vi "VSG25A_StepSweep.vi"(0 "Device Handle In":i32, 1 "Run as Subpanel":bool, 2 "RampSweep Cluster In":T1={"Start Freq"=990.0, "Stop Freq"=1010.0, "Start Hz"=2, "Stop Hz"=2, "Sweep Time"=10.0, "Amplitude"=-80.0, "Sweep Factor (sec)"=5} {"Sweep Factor (sec)" items=["tera", "giga", "Mega", "kilo", "unity", "milli", "micro", "nano", "pico"]; "Start Hz" items=["Hz", "kHz", "MHz", "GHz"]; "Stop Hz" items=["Hz", "kHz", "MHz", "GHz"]}, 3 "Error In":errorcluster) -> (5 "Device Handle Out":i32, 6 "RampSweep Cluster Out":T1 {"Sweep Factor (sec)" items=["tera", "giga", "Mega", "kilo", "unity", "milli", "micro", "nano", "pico"]; "Start Hz" items=["Hz", "kHz", "MHz", "GHz"]; "Stop Hz" items=["Hz", "kHz", "MHz", "GHz"]}, 7 "Error Out":errorcluster)   [LabVIEW 2014]
uses:
  Controls/Frequency Hertz.ctl
  Controls/Sweep Cluster.ctl
  Controls/Factor Control.ctl
  Controls/Ramp Sweep Write Steps.ctl
  sg_lib/VSG25A.lvlib
panel:
  in  "Sweep Factor \n(Seconds)":T3 items=["tera", "giga", "Mega", "kilo", "unity", "milli", "micro", "nano", "pico"]
  out "Frequency Span":dbl
  in  "Stop":bool
  out "Device Selected":bool
  in  "Sweep Time":dbl
  in  "Stop Hz":T2 items=["Hz", "kHz", "MHz", "GHz"]
  in  "Stop Frequency":dbl
  in  "RF On":bool
  in  "Start Hz":T2 items=["Hz", "kHz", "MHz", "GHz"]
  in  "Amplitude (dBm)":dbl
  in  "Start Frequency":dbl
  # "Step Sweep"
  # "(<= 10/Span)"
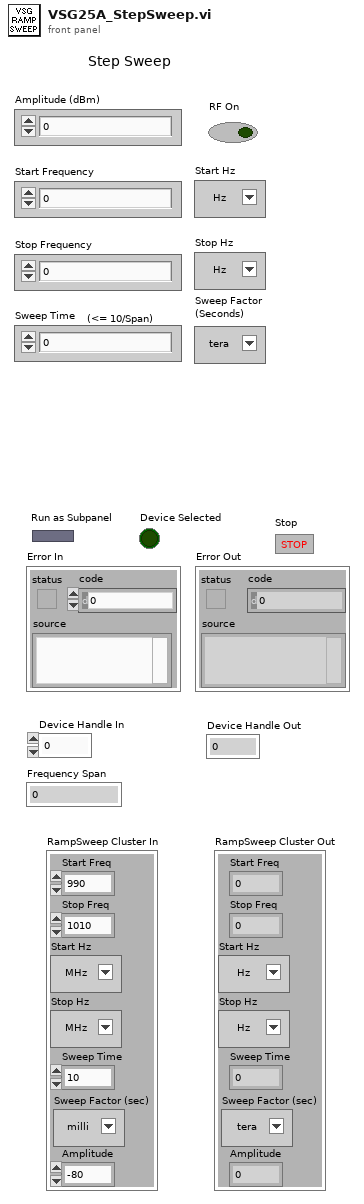
[diagram p1: front panel]
types:
  T1 = typedef "Sweep Cluster.ctl" = cluster{"Start Freq":dbl, "Stop Freq":dbl, "Start Hz":T2, "Stop Hz":T2, "Sweep Time":dbl, "Amplitude":dbl, "Sweep Factor (sec)":T3}
  T2 = typedef "Frequency Hertz.ctl" = u16
  T3 = typedef "Factor Control.ctl" = u16
  T4 = enum16{"Init", "Proc Events", "Write VSG25", "Exit"}
  T5 = enum32{"Bad", "Idle", "Run top level", "Running"}
  T6 = typedef "Ramp Sweep Write Steps.ctl" = enum16{"Check Amplitude", "Check Start Freq", "Check Stop Freq", "Check Sweep Time", "Calc Freq Span", "Stop RF", "Set Freq And Amp", "Set Sweep", "Finish", ""}
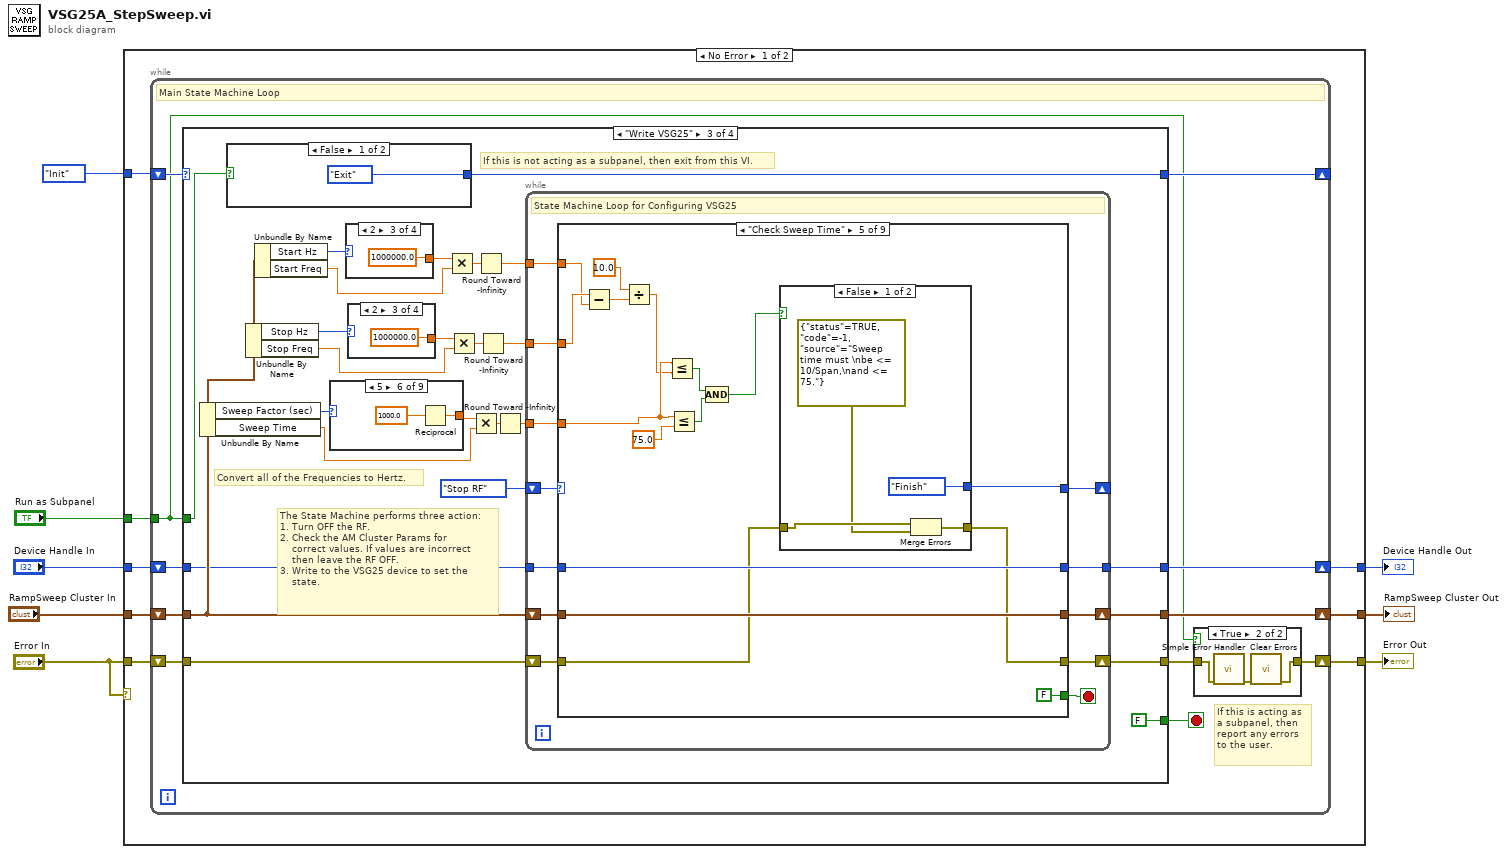
[diagram p0: block diagram]
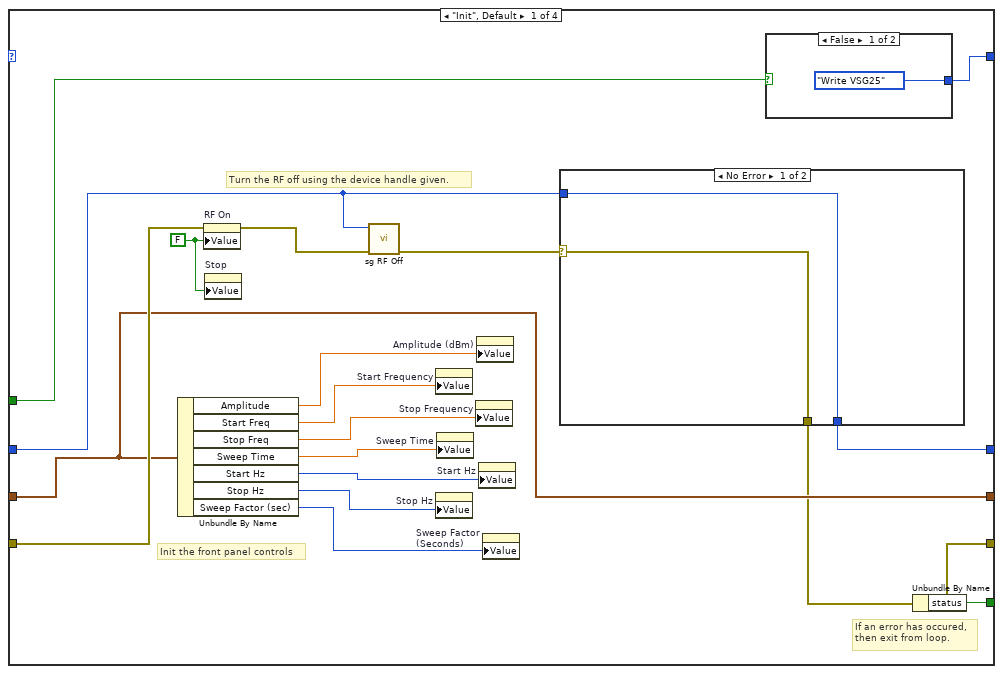
[diagram p3: hidden frame]
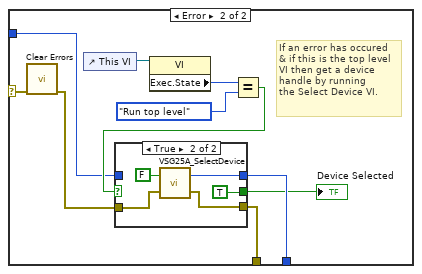
[diagram p4: hidden frame]
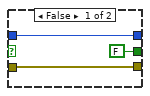
[diagram p5: hidden frame]
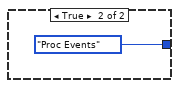
[diagram p6: hidden frame]
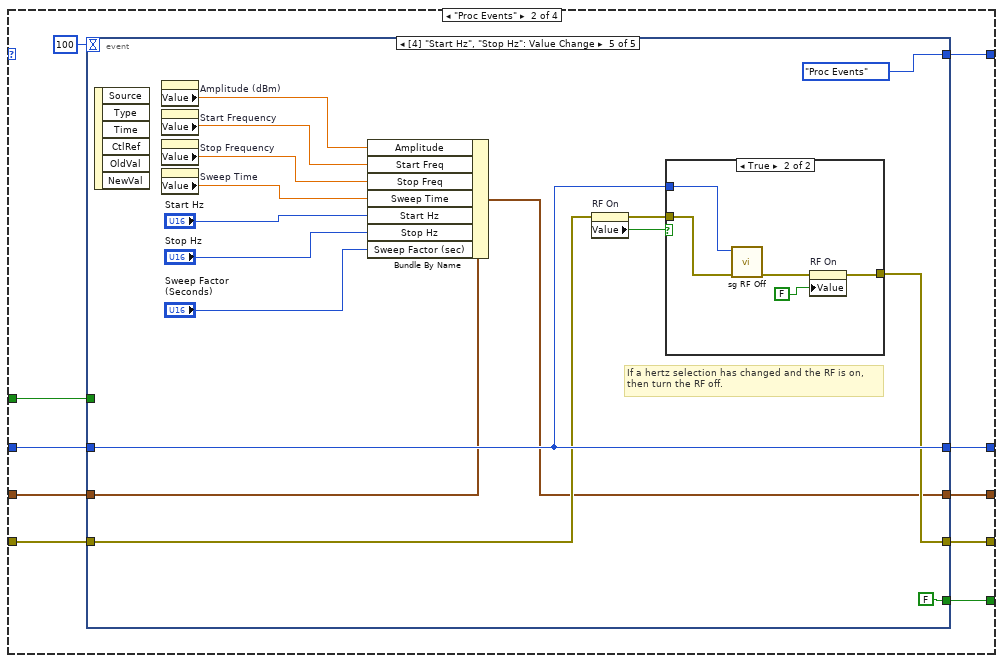
[diagram p7: hidden frame]
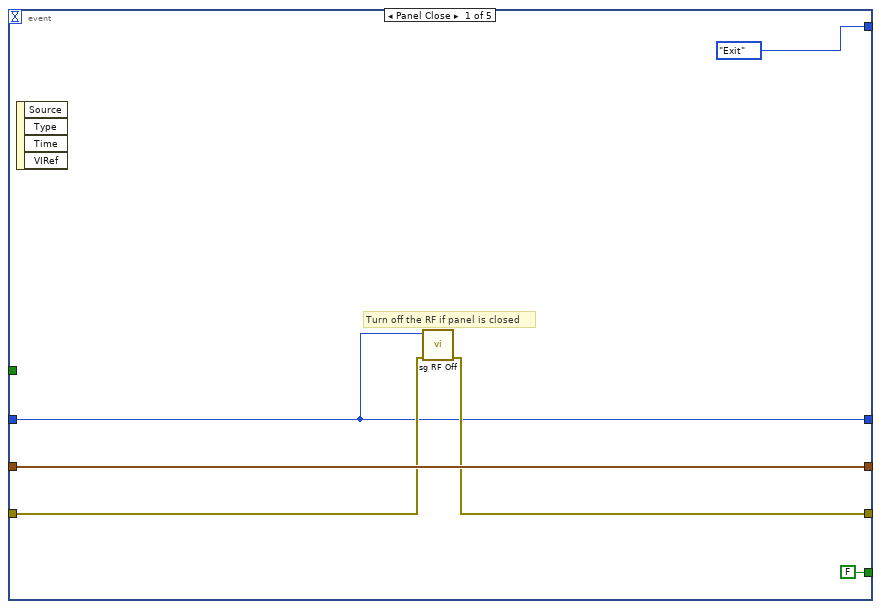
[diagram p8: hidden frame]
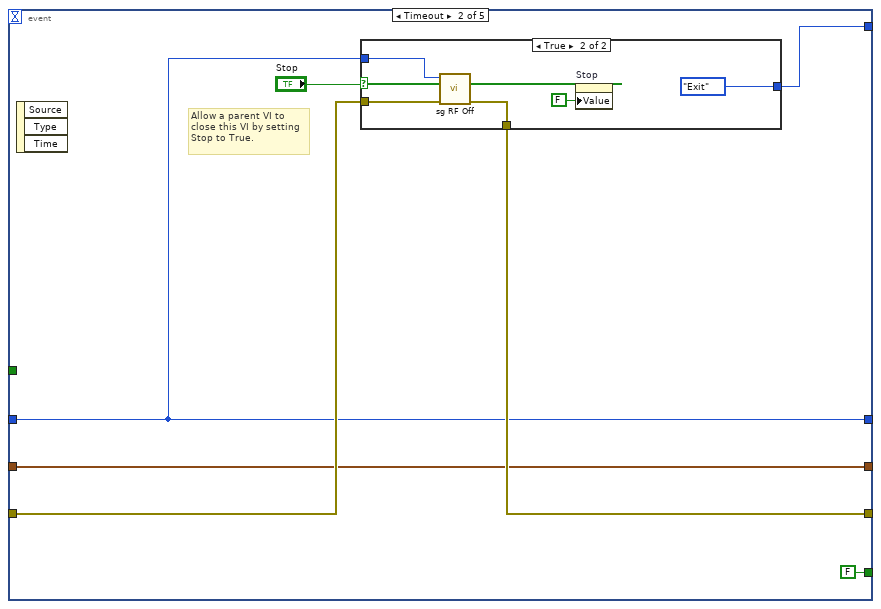
[diagram p9: hidden frame]
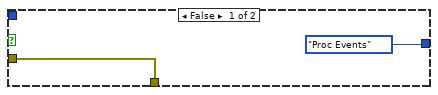
[diagram p10: hidden frame]
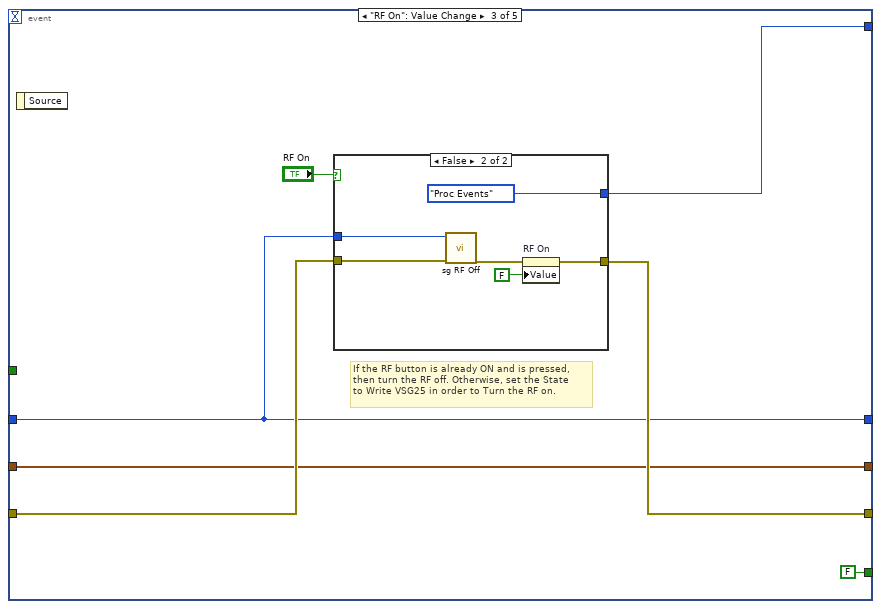
[diagram p11: hidden frame]
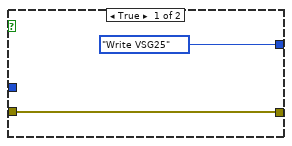
[diagram p12: hidden frame]
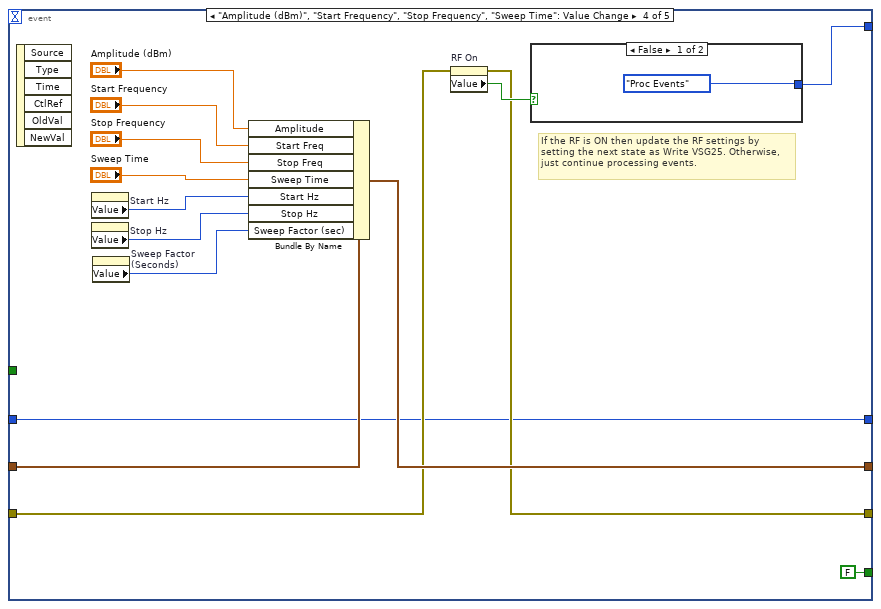
[diagram p13: hidden frame]
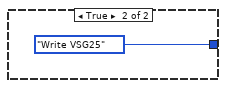
[diagram p14: hidden frame]
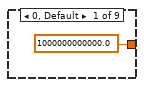
[diagram p16: hidden frame]
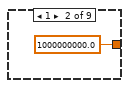
[diagram p17: hidden frame]
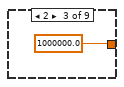
[diagram p18: hidden frame]
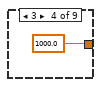
[diagram p19: hidden frame]
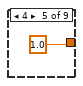
[diagram p20: hidden frame]
diagram:
  n1 = case shown="No Error" "Error In" {
    tunnel: "Error In" -> [w12 w360]
    tunnel: T4."Init" -> [w16 _]
    tunnel: "Run as Subpanel" -> [w15 _]
    tunnel: "Device Handle In" -> [w14 w358]
    tunnel: "RampSweep Cluster In" -> [w13 w359]
    tunnel: [w11 w360] -> w4
    tunnel: [w10 w359] -> w2
    tunnel: [w9 w358] -> w3
    frame No Error {
      n2 = while {
        shift-right: [w26] -> _
        shift-left: w16 -> [w27]
        tunnel: w15 -> [w17]
        shift-right: [w18] -> w11
        shift-left: w12 -> [w23]
        shift-right: [w21] -> w10
        shift-left: w13 -> [w24]
        shift-right: [w20] -> w9
        shift-left: w14 -> [w25]
        stop <- w22 stop-if-true
        # "If this is acting as \na subpanel, then\nreport any errors\nto the user."
        # "Main State Machine Loop"
        n3 = case shown="\"Write VSG25\"" w27 {
          selector: w27 -> [_ _ _ w353]
          tunnel: [w42 w74 w161 w353] -> w26
          tunnel: w17 -> [w45 w78 w160 _]
          tunnel: w25 -> [w36 w79 w166 w348]
          tunnel: w24 -> [w43 w80 w167 w349]
          tunnel: w23 -> [w44 w81 w171 w350]
          tunnel: [w41 w75 FALSE TRUE] -> w22
          tunnel: [w37 w73 w165 w351] -> w19
          tunnel: [w43 w77 w164 w349] -> w21
          tunnel: [w38 w76 w163 w348] -> w20
          frame "Init", Default {
            w35 = FALSE ("RF On")
            # "Init the front panel controls"
            # "Turn the RF off using the device handle given."
            # "If an error has occured,\nthen exit from loop."
            n4 = Unbundle By Name(w43) -> ("Amplitude"=w49:dbl, "Start Freq"=w48:dbl, "Stop Freq"=w47:dbl, "Sweep Time"=w46:dbl, "Start Hz"=w34:T2, "Stop Hz"=w33:T2, "Sweep Factor (sec)"=w32:T3)
            n5 = property on="RF On" class="Bool (strict)"(error in=w44, "Value"=w35) -> (error out=w40:errorcluster)  [unwired: 1 in, 1 out]
            n6 = property on="Stop" class="Bool (strict)"("Value"=w35) -> ()  [unwired: 2 in, 2 out]
            n7 = call "sg RF Off.vi"("error in (no error)"=w40, "device"=w36) -> ("error out"=w39:errorcluster)  [unwired: 8 in, 1 out]
            n8 = property on="Start Frequency" class="DigNum (strict)"("Value"=w48) -> ()  [unwired: 2 in, 2 out]
            n9 = property on="Stop Hz" class="Ring (strict)"("Value"=w33) -> ()  [unwired: 2 in, 2 out]
            n10 = property on="Sweep Time" class="DigNum (strict)"("Value"=w46) -> ()  [unwired: 2 in, 2 out]
            n11 = property on="Stop Frequency" class="DigNum (strict)"("Value"=w47) -> ()  [unwired: 2 in, 2 out]
            n12 = property on="Amplitude (dBm)" class="DigNum (strict)"("Value"=w49) -> ()  [unwired: 2 in, 2 out]
            n13 = property on="Start Hz" class="Ring (strict)"("Value"=w34) -> ()  [unwired: 2 in, 2 out]
            n14 = property on="Sweep Factor \n(Seconds)" class="Ring (strict)"("Value"=w32) -> ()  [unwired: 2 in, 2 out]
            n15 = case shown="No Error" w39 {
              selector: w39 -> [w50 w57]
              tunnel: [w51 w55] -> w38
              tunnel: [w50 w54] -> w37
              tunnel: w36 -> [w51 w53]
              frame No Error {
              }
              frame Error {
                # "If an error has occured\n& if this is the top level\nVI then get a device\nhandle by running \nthe Select Device VI."
                n16 = call <vilib>:"Clear Errors.vi"("error in (no error)"=w57) -> ("error out"=w56:errorcluster)  [unwired: 5 in, 1 out]
                n17 = control-ref of="This VI"() -> (w61:refnum<vi>)
                n18 = property class="VI"(reference=w61) -> ("Exec.State"=w60:T5)  [unwired: 1 in, 2 out]
                n19 = Equal?(x=w60, y=T5."Run top level" ("Execution:State 2")) -> (x = y?=w58:bool)
                n20 = case shown="True" w58 {
                  tunnel: [w64 w69] -> w55
                  tunnel: w53 -> [w64 _]
                  tunnel: w56 -> [w63 w67]
                  tunnel: [w63 w66] -> w54
                  tunnel: [FALSE TRUE] -> w52
                  frame False {
                  }
                  frame True {
                    n21 = call "VSG25A_SelectDevice.vi"("ErrorIn"=w67, "AutoSel"=FALSE) -> ("ErrorOut"=w66:errorcluster, "deviceHandle"=w69:i32)
                  }
                }
                "Device Selected" <- w52
              }
            }
            n22 = case shown="False" w45 {
              tunnel: [T4."Write VSG25" T4."Proc Events"] -> w42
              frame False {
              }
              frame True {
              }
            }
            n23 = Unbundle By Name(w37) -> ("status"=w41:bool)
          }
          frame "Proc Events" {
            n24 = event shown="[4] \"Start Hz\", \"Stop Hz\": Value Change" {
              selector: _ -> [_ _ _ _ _]
              dyn-events: _ -> [_ _ _ _ _]
              timeout: 100 -> [_ _ _ _ _]
              tunnel: w81 -> [w84 w91 w107 w123 w145]
              tunnel: w80 -> [w85 w89 w105 w131 w144]
              tunnel: w79 -> [w82 w88 w104 w121 w147]
              tunnel: w78 -> [_ _ _ _ _]
              tunnel: [w83 w90 w106 w122 w146] -> w73
              tunnel: [w85 w89 w105 w130 w143] -> w77
              tunnel: [w82 w88 w104 w121 w147] -> w76
              tunnel: [FALSE FALSE FALSE FALSE FALSE] -> w75
              tunnel: [T4."Exit" w92 w103 w124 T4."Proc Events"] -> w74
              event Panel Close {
                # "Turn off the RF if panel is closed"
                n25 = event-data() -> ()  [unwired: 1 in, 4 out]
                n26 = call "sg RF Off.vi"("error in (no error)"=w84, "device"=w82) -> ("error out"=w83:errorcluster)  [unwired: 8 in, 1 out]
              }
              event Timeout {
                # "Allow a parent VI to \nclose this VI by setting\nStop to True."
                n27 = event-data() -> ()  [unwired: 1 in, 3 out]
                n28 = case shown="True" "Stop" {
                  tunnel: [T4."Proc Events" T4."Exit"] -> w92
                  tunnel: w91 -> [w95 w100]
                  tunnel: [w95 w99] -> w90
                  tunnel: w88 -> [_ w98]
                  frame False {
                  }
                  frame True {
                    n29 = call "sg RF Off.vi"("error in (no error)"=w100, "device"=w98) -> ("error out"=w99:errorcluster)  [unwired: 8 in, 1 out]
                    n30 = property on="Stop" class="Bool (strict)"("Value"=FALSE ("Stop")) -> ()  [unwired: 2 in, 2 out]
                  }
                }
              }
              event "RF On": Value Change {
                # "If the RF button is already ON and is pressed, \nthen turn the RF off. Otherwise, set the State\nto Write VSG25 in order to Turn the RF on."
                n31 = event-data() -> ()  [unwired: 1 in, 1 out]
                n32 = case shown="False" "RF On" {
                  tunnel: [w109 w114] -> w106
                  tunnel: w107 -> [w109 w116]
                  tunnel: w104 -> [_ w115]
                  tunnel: [T4."Write VSG25" T4."Proc Events"] -> w103
                  frame True {
                  }
                  frame False {
                    n33 = call "sg RF Off.vi"("error in (no error)"=w116, "device"=w115) -> ("error out"=w113:errorcluster)  [unwired: 8 in, 1 out]
                    n34 = property on="RF On" class="Bool (strict)"(error in=w113, "Value"=FALSE ("RF On")) -> (error out=w114:errorcluster)  [unwired: 1 in, 1 out]
                  }
                }
              }
              event "Amplitude (dBm)", "Start Frequency", "Stop Frequency", "Sweep Time": Value Change {
                # "If the RF is ON then update the RF settings by\nsetting the next state as Write VSG25. Otherwise,\njust continue processing events."
                n35 = event-data() -> ()  [unwired: 1 in, 6 out]
                n36 = property on="Start Hz" class="Ring (strict)"() -> ("Value"=w119:T2)  [unwired: 2 in, 2 out]
                n37 = property on="Stop Hz" class="Ring (strict)"() -> ("Value"=w118:T2)  [unwired: 2 in, 2 out]
                n38 = property on="Sweep Factor \n(Seconds)" class="Ring (strict)"() -> ("Value"=w117:T3)  [unwired: 2 in, 2 out]
                n39 = Bundle By Name(cluster=w131, "Amplitude"="Amplitude (dBm)", "Start Freq"="Start Frequency", "Stop Freq"="Stop Frequency", "Sweep Time"="Sweep Time", "Start Hz"=w119, "Stop Hz"=w118, "Sweep Factor (sec)"=w117) -> (w130:T1)
                n40 = property on="RF On" class="Bool (strict)"(error in=w123) -> (error out=w122:errorcluster, "Value"=w125:bool)  [unwired: 1 in, 1 out]
                n41 = case shown="False" w125 {
                  tunnel: [T4."Proc Events" T4."Write VSG25"] -> w124
                  frame False {
                  }
                  frame True {
                  }
                }
              }
              event Value Change {
                # "If a hertz selection has changed and the RF is on,\nthen turn the RF off."
                n42 = event-data() -> ()  [unwired: 1 in, 6 out]
                n43 = property on="Amplitude (dBm)" class="DigNum (strict)"() -> ("Value"=w142:dbl)  [unwired: 2 in, 2 out]
                n44 = property on="Start Frequency" class="DigNum (strict)"() -> ("Value"=w141:dbl)  [unwired: 2 in, 2 out]
                n45 = property on="Stop Frequency" class="DigNum (strict)"() -> ("Value"=w140:dbl)  [unwired: 2 in, 2 out]
                n46 = property on="Sweep Time" class="DigNum (strict)"() -> ("Value"=w139:dbl)  [unwired: 2 in, 2 out]
                n47 = Bundle By Name(cluster=w144, "Amplitude"=w142, "Start Freq"=w141, "Stop Freq"=w140, "Sweep Time"=w139, "Start Hz"="Start Hz", "Stop Hz"="Stop Hz", "Sweep Factor (sec)"="Sweep Factor \n(Seconds)") -> (w143:T1)
                n48 = property on="RF On" class="Bool (strict)"(error in=w145) -> (error out=w149:errorcluster, "Value"=w148:bool)  [unwired: 1 in, 1 out]
                n49 = case shown="True" w148 {
                  tunnel: [w150 w151] -> w146
                  tunnel: w149 -> [w150 w155]
                  tunnel: w147 -> [_ w154]
                  frame False {
                  }
                  frame True {
                    n50 = call "sg RF Off.vi"("error in (no error)"=w155, "device"=w154) -> ("error out"=w152:errorcluster)  [unwired: 8 in, 1 out]
                    n51 = property on="RF On" class="Bool (strict)"(error in=w152, "Value"=FALSE ("RF On")) -> (error out=w151:errorcluster)  [unwired: 1 in, 1 out]
                  }
                }
              }
            }
          }
          frame "Write VSG25" {
            # "If this is not acting as a subpanel, then exit from this VI."
            # "Convert all of the Frequencies to Hertz."
            # "The State Machine performs three action:\n1. Turn OFF the RF.\n2. Check the AM Cluster Params for \n    correct values. If values are incorrect\n    then leave the RF OFF.\n3. Write to the VSG25 device to set the\n    state."
            n52 = Unbundle By Name(w167) -> ("Sweep Factor (sec)"=w159:T3, "Sweep Time"=w158:dbl)
            n53 = case shown="False" w160 {
              tunnel: [T4."Exit" T4."Proc Events"] -> w161
              frame False {
              }
              frame True {
              }
            }
            n54 = Unbundle By Name(w167) -> ("Stop Hz"=w174:T2, "Stop Freq"=w176:dbl)
            n55 = Unbundle By Name(w167) -> ("Start Hz"=w179:T2, "Start Freq"=w177:dbl)
            n56 = case shown="5" w159 {
              tunnel: [1000000000000.0 1000000000.0 ("y") 1000000.0 ("y") 1000.0 ("y") 1.0 ("y") w187 w189 w191 w193] -> w157
              frame 0, Default {
              }
              frame 1 {
              }
              frame 2 {
              }
              frame 3 {
              }
              frame 4 {
              }
              frame 5 {
                n57 = Reciprocal(x=1000.0 ("y")) -> (1/x=w187:dbl)
              }
              frame 6 {
                n58 = Reciprocal(x=1000000.0 ("y")) -> (1/x=w189:dbl)
              }
              frame 7 {
                n59 = Reciprocal(x=1000000000.0 ("y")) -> (1/x=w191:dbl)
              }
              frame 8 {
                n60 = Reciprocal(x=1000000000000.0) -> (1/x=w193:dbl)
              }
            }
            n61 = case shown="2" w179 {
              tunnel: [1.0 ("y") 1000.0 ("y") 1000000.0 ("y") 1000000000.0 ("y")] -> w178
              frame 0, Default {
              }
              frame 1 {
              }
              frame 2 {
              }
              frame 3 {
              }
            }
            n62 = case shown="2" w174 {
              tunnel: [1.0 ("y") 1000.0 ("y") 1000000.0 ("y") 1000000000.0 ("y")] -> w175
              frame 0, Default {
              }
              frame 1 {
              }
              frame 2 {
              }
              frame 3 {
              }
            }
            n63 = Multiply(x=w178, y=w177) -> (x*y=w180:dbl)
            n64 = Multiply(x=w175, y=w176) -> (x*y=w173:dbl)
            n65 = Multiply(x=w157, y=w158) -> (x*y=w172:dbl)
            n66 = Round Toward -Infinity(1:w180) -> (0:w170:dbl)
            n67 = Round Toward -Infinity(1:w173) -> (0:w169:dbl)
            n68 = Round Toward -Infinity(1:w172) -> (0:w168:dbl)
            n69 = while {
              tunnel: w170 -> [w210]
              tunnel: w169 -> [w209]
              tunnel: w168 -> [w208]
              tunnel: w166 -> [w206]
              tunnel: [w203] -> w163
              shift-right: [w205] -> w165
              shift-left: w171 -> [w211]
              shift-right: [w204] -> w164
              shift-left: w167 -> [w207]
              shift-right: [w200] -> _
              shift-left: Ramp_Sweep_Write_Steps."Stop RF" -> [w201]
              stop <- w202 stop-if-true
              # "State Machine Loop for Configuring VSG25"
              n70 = case shown="\"Check Sweep Time\"" w201 {
                selector: w201 -> [_ _ _ _ _ _ _ _ w335]
                tunnel: w211 -> [w217 w220 w257 w275 w297 w310 w325 w334 w336]
                tunnel: w210 -> [_ _ w248 _ w290 w309 w317 _ _]
                tunnel: w209 -> [_ _ w247 w269 w291 w308 _ _ _]
                tunnel: w208 -> [_ _ _ _ w287 _ _ w327 _]
                tunnel: w207 -> [w215 w224 w258 w277 w299 w314 w323 w332 w337]
                tunnel: w206 -> [w214 w222 w259 w276 w298 w313 w322 w331 w338]
                tunnel: [w216 w219 w256 w274 w296 w310 w324 w333 w336] -> w205
                tunnel: [w215 w223 w258 w277 w299 w314 w323 w332 w337] -> w204
                tunnel: [w214 w222 w259 w276 w298 w313 w322 w331 w338] -> w203
                tunnel: [FALSE FALSE FALSE FALSE FALSE FALSE FALSE FALSE TRUE] -> w202
                tunnel: [Ramp_Sweep_Write_Steps."Check Amplitude" w218 w250 w267 w292 Ramp_Sweep_Write_Steps."Set Freq And Amp" Ramp_Sweep_Write_Steps."Set Sweep" Ramp_Sweep_Write_Steps."Finish" w335] -> w200
                frame "Stop RF", Default {
                  n71 = call "sg RF Off.vi"("error in (no error)"=w217, "device"=w214) -> ("error out"=w216:errorcluster)  [unwired: 8 in, 1 out]
                }
                frame "Check Amplitude" {
                  n72 = Unbundle By Name(w224) -> ("Amplitude"=w230:dbl)
                  n73 = Less Or Equal?(x=w230, y=10.0) -> (x <= y?=w226:bool)
                  n74 = Greater Or Equal?(x=w230, y=-80.0) -> (x >= y?=w229:bool)
                  n75 = And(x=w226, y=w229) -> (x .and. y?=w225:bool)
                  n76 = case shown="True" w225 {
                    tunnel: w229 -> [w240 _]
                    tunnel: w230 -> [_ w245]
                    tunnel: w224 -> [w237 w244]
                    tunnel: [w236 w243] -> w223
                    tunnel: w220 -> [w234 w242]
                    tunnel: [w232 w242] -> w219
                    tunnel: [Ramp_Sweep_Write_Steps."Finish" Ramp_Sweep_Write_Steps."Check Start Freq"] -> w218
                    frame False {
                      n77 = Select(t=10.0, s=w240, f=-80.0) -> (s? t:f=w235:dbl)
                      n78 = Bundle By Name(cluster=w237, "Start Freq"=w235) -> (w236:T1)
                      n79 = property on="Amplitude (dBm)" class="DigNum (strict)"("Value"=w235) -> ()  [unwired: 2 in, 2 out]
                      n80 = Merge Errors(w234, errorcluster {"status"=TRUE, "code"=-1, "source"="Invalid Amplitude.\nValue must be between\n-80 dBm and 10 dBm."} ("error constant")) -> (w232:errorcluster)
                    }
                    frame True {
                      n81 = Round Toward -Infinity(1:w245) -> (0:w246:dbl)
                      n82 = Bundle By Name(cluster=w244, "Amplitude"=w246) -> (w243:T1)
                    }
                  }
                }
                frame "Check Start Freq" {
                  n83 = Greater Or Equal?(x=w248, y=80000000.0) -> (x >= y?=w254:bool)
                  n84 = Less?(x=w248, y=w247) -> (x < y?=w249:bool)
                  n85 = Less Or Equal?(x=w248, y=2500000000.0) -> (x <= y?=w255:bool)
                  n86 = Compound Arithmetic op=AND(w254, w249, w255) -> (w251:bool)
                  n87 = case shown="True" w251 {
                    tunnel: w257 -> [w263 w266]
                    tunnel: [w264 w266] -> w256
                    tunnel: [Ramp_Sweep_Write_Steps."Finish" Ramp_Sweep_Write_Steps."Check Stop Freq"] -> w250
                    frame False {
                      n88 = Merge Errors(w263, errorcluster {"status"=TRUE, "code"=-1, "source"="Start frequency must \nbe greater than 80 MHz,\nless than 2.5 GHz and \nless than stop frequency."} ("error constant")) -> (w264:errorcluster)
                    }
                    frame True {
                    }
                  }
                }
                frame "Check Stop Freq" {
                  n89 = Greater Or Equal?(x=w269, y=80000000.0) -> (x >= y?=w272:bool)
                  n90 = Less Or Equal?(x=w269, y=2500000000.0) -> (x <= y?=w273:bool)
                  n91 = Compound Arithmetic op=AND(w272, w273) -> (w268:bool)
                  n92 = case shown="True" w268 {
                    tunnel: w275 -> [w282 w284]
                    tunnel: [w280 w284] -> w274
                    tunnel: [Ramp_Sweep_Write_Steps."Finish" Ramp_Sweep_Write_Steps."Check Sweep Time"] -> w267
                    frame False {
                      n93 = Merge Errors(w282, errorcluster {"status"=TRUE, "code"=-1, "source"="Stop frequency must \nbe greater than 80 MHz,\nand less than 2.5 GHz."} ("error constant")) -> (w280:errorcluster)
                    }
                    frame True {
                    }
                  }
                }
                frame "Check Sweep Time" {
                  n94 = Subtract(x=w291, y=w290) -> (x-y=w288:dbl)
                  n95 = Divide(x=10.0, y=w288) -> (x/y=w286:dbl)
                  n96 = Less Or Equal?(x=w287, y=w286) -> (x <= y?=w285:bool)
                  n97 = Less Or Equal?(x=w287, y=75.0) -> (x <= y?=w295:bool)
                  n98 = Compound Arithmetic op=AND(w285, w295) -> (w293:bool)
                  n99 = case shown="False" w293 {
                    tunnel: w297 -> [w303 w306]
                    tunnel: [w304 w306] -> w296
                    tunnel: [Ramp_Sweep_Write_Steps."Finish" Ramp_Sweep_Write_Steps."Calc Freq Span"] -> w292
                    frame False {
                      n100 = Merge Errors(w303, errorcluster {"status"=TRUE, "code"=-1, "source"="Sweep time must \nbe <= 10/Span,\nand <= 75."} ("error constant")) -> (w304:errorcluster)
                    }
                    frame True {
                    }
                  }
                }
                frame "Calc Freq Span" {
                  n101 = Subtract(x=w308, y=w309) -> (x-y=→"Frequency Span":dbl)
                }
                frame "Set Freq And Amp" {
                  # "Specify the center frequency of the freq span."
                  n102 = property on="Frequency Span" class="DigNum (strict)"() -> ("Value"=w318:dbl)  [unwired: 2 in, 2 out]
                  n103 = Divide(x=w318, y=2.0) -> (x/y=w320:dbl)
                  n104 = Unbundle By Name(w323) -> ("Amplitude"=w326:dbl)
                  n105 = Add(x=w317, y=w320) -> (x+y=w316:dbl)
                  n106 = call "sg Set Frequency Amplitude.vi"("error in (no error)"=w325, "amplitude"=w326, "frequency"=w316, "device"=w322) -> ("error out"=w324:errorcluster)  [unwired: 6 in, 1 out]
                }
                frame "Set Sweep" {
                  n107 = property on="Frequency Span" class="DigNum (strict)"() -> ("Value"=w328:dbl)  [unwired: 2 in, 2 out]
                  n108 = call "sg Set Sweep.vi"("error in (no error)"=w334, "span"=w328, "time"=w327, "device"=w331) -> ("error out"=w333:errorcluster)  [unwired: 6 in, 1 out]
                }
                frame "Finish" {
                  # "If no errors have occured, then indicate that the RF is ON."
                  n109 = case shown="Error" w336 {
                    tunnel: [TRUE FALSE] -> w340
                    frame No Error {
                    }
                    frame Error {
                    }
                  }
                  n110 = property on="RF On" class="Bool (strict)"("Value"=w340) -> ()  [unwired: 2 in, 2 out]
                }
              }
            }
          }
          frame "Exit" {
            # "If a device handle was\nacquired using the \nSelect Device VI, then\nclose the handle \nbefore exiting."
            n111 = local read "Device Selected"() -> (w347:bool)
            n112 = case shown="True" w347 {
              tunnel: w348 -> [_ w357]
              tunnel: w350 -> [w354 w356]
              tunnel: [w354 w355] -> w351
              frame False {
              }
              frame True {
                n113 = call "sg Close Device.vi"("error in (no error)"=w356, "device"=w357) -> ("error out"=w355:errorcluster)  [unwired: 8 in, 1 out]
              }
            }
          }
        }
        n114 = case shown="True" w17 {
          tunnel: w19 -> [w28 w30]
          tunnel: [w28 w31] -> w18
          frame False {
          }
          frame True {
            n115 = call <vilib>:"Simple Error Handler.vi"("error in (no error)"=w30) -> ("error out"=w29:errorcluster)  [unwired: 4 in, 4 out]
            n116 = call <vilib>:"Clear Errors.vi"("error in (no error)"=w29) -> ("error out"=w31:errorcluster)  [unwired: 5 in, 1 out]
          }
        }
      }
    }
    frame Error {
    }
  }
  "Error Out" <- w4
  "Device Handle Out" <- w3
  "RampSweep Cluster Out" <- w2
